vi "In_S2F41.vi"(8 "error in (no error)":errorcluster, 11 "S2 Message Class in":refnum<class "S2 Message Class.lvclass">) -> (0 "error out":errorcluster, 1 "OK?":bool, 2 "S2F41":T1, 3 "S2 Message Class out":refnum<class "S2 Message Class.lvclass">)   [LabVIEW 2020, in "SECS Communication.lvlib" / "S2 Message Class.lvclass"]
uses:
  S2 Message Class.lvclass
  D:/Dropbox/SECS/SECS_GEM v1.0.6/Com/SECS Communication/SECS-II Class/SECS-II Class.lvclass
  S2F41.ctl
  SECS-II Class/SECS-II Class.lvclass/SECS-II Class.ctl
  SECS-II Class/Variant To Data_ASCII.vi
  SECS-II Class/SECS-II Class.lvclass
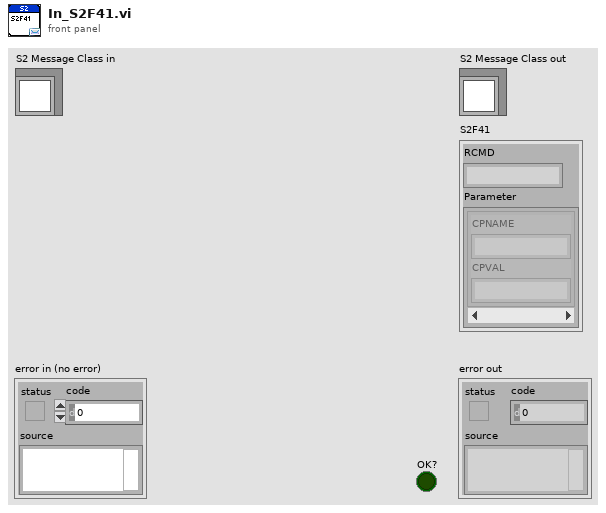
[diagram p1: front panel]
types:
  T1 = typedef "SECS Communication.lvlib/S2 Message Class.lvclass/S2F41.ctl" = cluster{"RCMD":string, "Parameter":cluster{"CPNAME":string, "CPVAL":string}[]}
  T2 = typedef "SECS Communication.lvlib/SECS-II Class.lvclass/Message Data.ctl" = cluster{"Index":i32, "Data Item Format":T3, "Format Code":T4, "Parent Index":i32, "Child Index":i32[], "Data":variant}
  T3 = typedef "SECS Communication.lvlib/SECS-II Class.lvclass/Data Item Format.ctl" = enum16{"Data Type", "Value"}
  T4 = typedef "SECS Communication.lvlib/SECS-II Class.lvclass/Format Code.ctl" = enum16{"L", "A", "B", "Boolean", "J", "I1", "I2", "I4", "I8", "U1", "U2", "U4", "U8", "F4", "F8", "Char"}
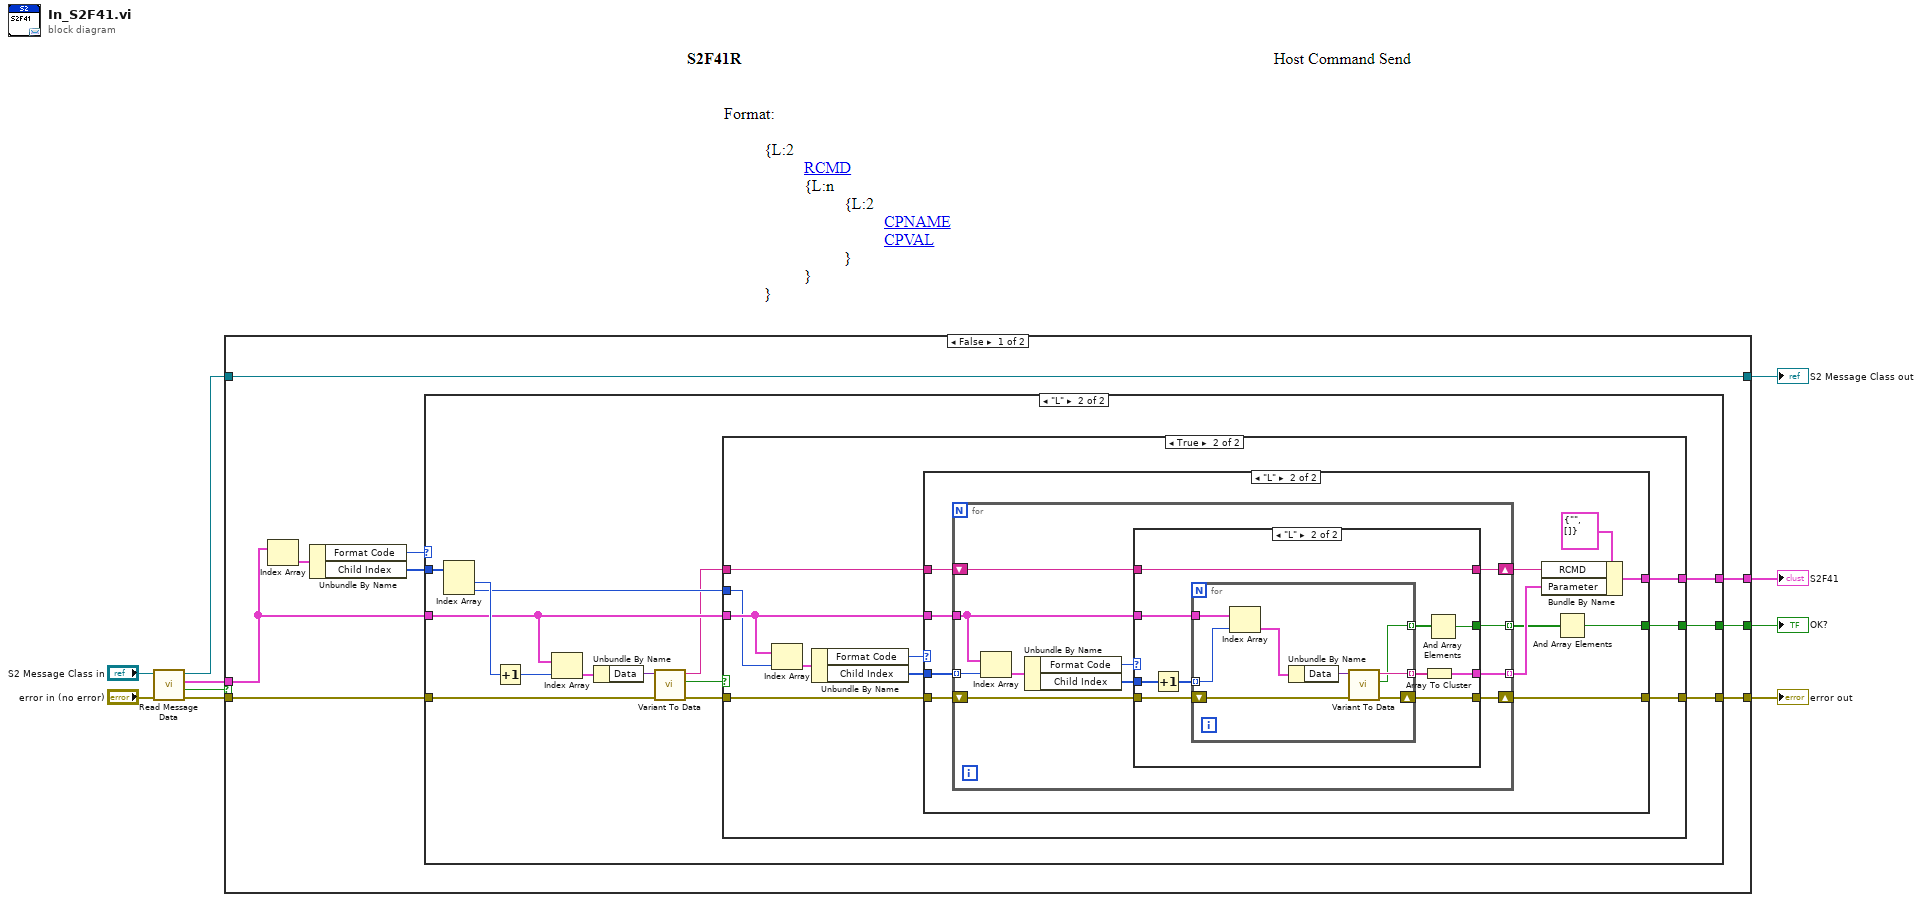
[diagram p0: block diagram]
diagram:
  n1 = call "Read Message Data.vi"("error in (no error)"="error in (no error)", "SECS-II Class in"="S2 Message Class in") -> ("error out"=w10:errorcluster, "Empty?"=w3:bool, "Message Data"=w9:T2[], "SECS-II Class out"=w2:refnum<class "S2 Message Class.lvclass">)  [unwired: 6 in]
  n2 = case shown="False" w3 {
    tunnel: w10 -> [w17 w89]
    tunnel: w9 -> [w16 _]
    tunnel: [w15 w89] -> w8
    tunnel: [w14 _] -> w7
    tunnel: [w12 _] -> w4
    tunnel: w2 -> [w11 w90]
    tunnel: [w11 w90] -> w1
    frame False {
      n3 = Index Array(array=w16) -> (element=w19:T2)  [unwired: 1 in]
      n4 = Unbundle By Name(w19) -> ("Format Code"=w13:T4, "Child Index"=w18:i32[])
      n5 = case shown="\"L\"" w13 {
        tunnel: w18 -> [_ w34]
        tunnel: w17 -> [w20 w31]
        tunnel: w16 -> [_ w27]
        tunnel: [w20 w24] -> w15
        tunnel: [_ w23] -> w14
        tunnel: [_ w21] -> w12
        frame Default {
        }
        frame "L" {
          n6 = Index Array(array=w34) -> (element #1=w33:i32, element #2=w26:i32)  [unwired: 2 in]
          n7 = Increment(x=w33) -> (x+1=w30:i32)
          n8 = Index Array(array=w27, index=w30) -> (element=w29:T2)
          n9 = Unbundle By Name(w29) -> ("Data"=w32:variant)
          n10 = call-poly "Variant To Data.vi"("error in (no error)"=w31, "Variant"=w32) -> ("error out"=w28:errorcluster, "OK?"=w22:bool, "Data"=w25:string)  [unwired: 7 in]
          n11 = case shown="True" w22 {
            tunnel: w28 -> [w35 w45]
            tunnel: w27 -> [_ w44]
            tunnel: w26 -> [_ w43]
            tunnel: w25 -> [_ w40]
            tunnel: [w35 w39] -> w24
            tunnel: [_ w38] -> w23
            tunnel: [_ w36] -> w21
            frame False {
            }
            frame True {
              n12 = Index Array(array=w44, index=w43) -> (element=w42:T2)
              n13 = Unbundle By Name(w42) -> ("Format Code"=w37:T4, "Child Index"=w41:i32[])
              n14 = case shown="\"L\"" w37 {
                tunnel: w45 -> [w46 w56]
                tunnel: w44 -> [_ w55]
                tunnel: w41 -> [_ w54]
                tunnel: w40 -> [_ w53]
                tunnel: [w46 w50] -> w39
                tunnel: [_ w49] -> w38
                tunnel: [_ w47] -> w36
                frame Default {
                }
                frame "L" {
                  n15 = for {
                    shift-right: [w63] -> w50
                    shift-left: w56 -> [w65]
                    tunnel: w55 -> [w64]
                    tunnel: w54 -> [w68] mode=indexing
                    shift-right: [w59] -> w52
                    shift-left: w53 -> [w60]
                    tunnel: [w62] -> w51 mode=indexing
                    tunnel: [w58] -> w48 mode=indexing
                    n16 = Index Array(array=w64, index=w68) -> (element=w67:T2)
                    n17 = Unbundle By Name(w67) -> ("Format Code"=w61:T4, "Child Index"=w66:i32[])
                    n18 = case shown="\"L\"" w61 {
                      tunnel: w66 -> [_ w80]
                      tunnel: w65 -> [w69 w79]
                      tunnel: w64 -> [_ w77]
                      tunnel: [w69 w76] -> w63
                      tunnel: [_ w74] -> w62
                      tunnel: w60 -> [w70 w73]
                      tunnel: [w70 w73] -> w59
                      tunnel: [_ w71] -> w58
                      frame Default {
                      }
                      frame "L" {
                        n19 = Increment(x=w80) -> (x+1=w78:i32[])
                        n20 = for {
                          shift-right: [w82] -> w76
                          shift-left: w79 -> [w85]
                          tunnel: w78 -> [w87] mode=indexing
                          tunnel: w77 -> [w88]
                          tunnel: [w83] -> w75 mode=indexing
                          tunnel: [w81] -> w72 mode=indexing
                          n21 = Index Array(array=w88, index=w87) -> (element=w86:T2)
                          n22 = Unbundle By Name(w86) -> ("Data"=w84:variant)
                          n23 = call-poly "Variant To Data.vi"("error in (no error)"=w85, "Variant"=w84) -> ("error out"=w82:errorcluster, "OK?"=w81:bool, "Data"=w83:string)  [unwired: 7 in]
                        }
                        n24 = Array To Cluster(array=w75) -> (cluster=w74:cluster{"[0]":string, "[1]":string})
                        n25 = And Array Elements(Boolean array=w72) -> (logical AND=w71:bool)
                      }
                    }
                  }
                  n26 = Bundle By Name(cluster=T1 {"RCMD"="", "Parameter"=[]} ("S2F41"), "RCMD"=w52, "Parameter"=w51) -> (w49:T1)
                  n27 = And Array Elements(Boolean array=w48) -> (logical AND=w47:bool)
                }
              }
            }
          }
        }
      }
    }
    frame True {
    }
  }
  "error out" <- w8
  "S2 Message Class out" <- w1
  "S2F41" <- w7
  "OK?" <- w4
